vi "Msg.Q.Release.vi"(8 "Error (in)":errorcluster, 11 "Msg.Refs":T1) -> (0 "Error (out)":errorcluster)   [LabVIEW 2023, in "MessagingModule.lvlib"]
doc: "This VI is used to destroy a queue of message and data."
uses:
  MessagingModule.lvlib
  Msg.Data.ctl
  Msg.Event.Ref.ctl
  Msg.Event.RegRef.ctl
  Msg.Q.Ref.ctl
  Msg.Refs.ctl
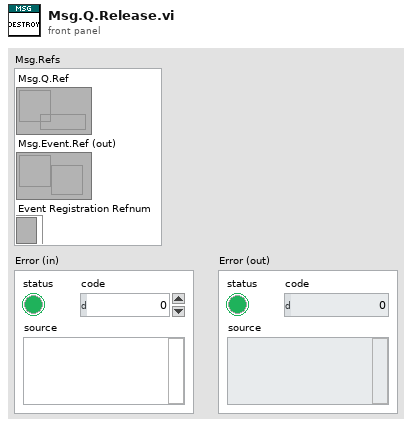
[diagram p1: front panel]
types:
  T1 = typedef "MessagingModule.lvlib/Msg.Refs.ctl" = cluster{"Msg.Q.Ref":T2, "Msg.Event.Ref (out)":T3, "Event Registration Refnum":T4}
  T2 = typedef "MessagingModule.lvlib/Msg.Q.Ref.ctl" = refnum<queue>
  T3 = typedef "MessagingModule.lvlib/Msg.Event.Ref.ctl" = refnum<user-event>
  T4 = typedef "MessagingModule.lvlib/Msg.Event.RegRef.ctl" = refnum<event-registration>
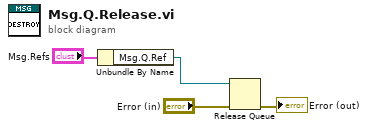
[diagram p0: block diagram]
diagram:
  n1 = Unbundle By Name("Msg.Refs") -> ("Msg.Q.Ref"=w1:T2)
  n2 = Release Queue(queue=w1, error in (no error)="Error (in)") -> (error out=→"Error (out)":errorcluster)  [unwired: 1 in, 2 out]
